vi "PathPlanner_TrigEventsSend.vi"(10 "Current Trig Events":T1[](array[typedef]) {"lastRobotPos"."Y" format="%14.3f"; "lastRobotPos"."X" format="%14.3f"; "markerPos"."Y" format="%14.3f"; "markerPos"."X" format="%14.3f"}) -> (2 "Past Trig EventMarkers":T1[](array[typedef]) {"lastRobotPos"."Y" format="%14.3f"; "lastRobotPos"."X" format="%14.3f"; "markerPos"."Y" format="%14.3f"; "markerPos"."X" format="%14.3f"}, 3 "Past Trig Events":string[](array[string]))   [LabVIEW 2023]
uses:
  <vilib>/Rock Robotics/WPI/ThirdParty/MJansen/PathPlanner/TypeDef/PathPlannerEventMarker.ctl
  <vilib>/Rock Robotics/WPI/ThirdParty/JAS_Junk/TrajLib/TypeDef/TRANSLATION2D.ctl
  <vilib>/Rock Robotics/WPI/ThirdParty/MJansen/PathPlanner/TypeDef/PathPlannerCommandUtil.ctl
  <vilib>/Rock Robotics/WPI/ThirdParty/MJansen/PathPlanner/ENum/PathPlanner_CommandUtilType_ENUM.ctl
  fee4c28f-3952-4fee-86c4-e7927070a504.vi
  <vilib>/Rock Robotics/WPI/ThirdParty/MJansen/PathPlanner/PathPlanner24.lvlib
  <vilib>/Rock Robotics/WPI/ThirdParty/JAS_Junk/TrajLib/Trajectory_Library.lvlib
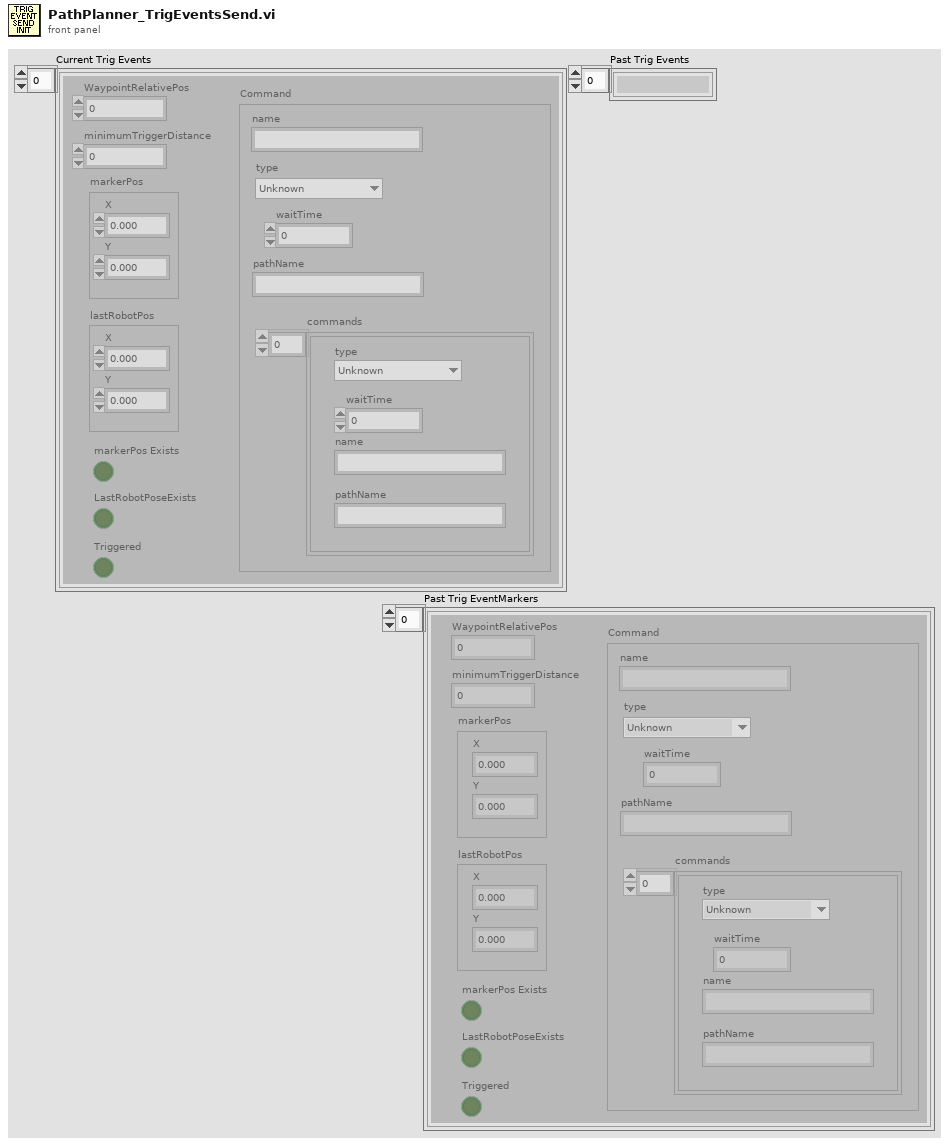
[diagram p1: front panel]
types:
  T1 = typedef "PathPlanner24.lvlib/PathPlannerEventMarker.ctl" = cluster{"WaypointRelativePos":dbl, "minimumTriggerDistance":dbl, "markerPos":T2, "lastRobotPos":T2, "Command":T3, "markerPos Exists":bool, "LastRobotPoseExists":bool, "Triggered":bool}
  T2 = typedef "Trajectory_Library.lvlib/TRANSLATION2D.ctl" = cluster{"X":dbl, "Y":dbl}
  T3 = typedef "PathPlanner24.lvlib/PathPlannerCommandUtil.ctl" = cluster{"waitTime":dbl, "name":string, "pathName":string, "commands":cluster{"type":T4, "waitTime":dbl, "name":string, "pathName":string}[], "type":T4}
  T4 = typedef "PathPlanner24.lvlib/PathPlanner_CommandUtilType_ENUM.ctl" = enum16{"Unknown", "Wait", "Named", "Path", "Sequential", "Parallel", "Race", "Deadline"}
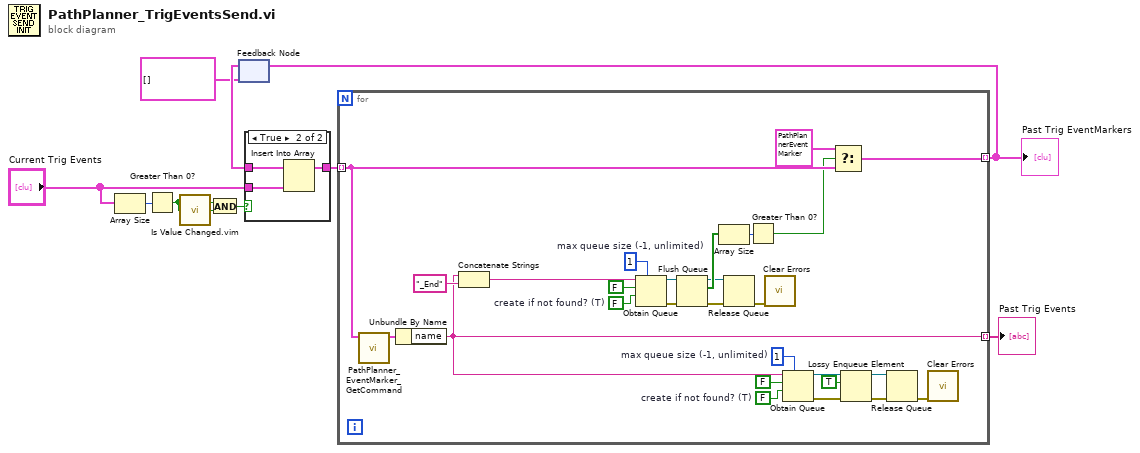
[diagram p0: block diagram]
diagram:
  n1 = Array Size(array="Current Trig Events") -> (size(s)=w3:i32)
  n2 = Greater Than 0?(x=w3) -> (x > 0?=w2:bool)
  n3 = call "Is Value Changed.vim"("value"=w2) -> ("changed or first call?"=w4:bool)
  n4 = And(x=w2, y=w4) -> (x .and. y?=w1:bool)
  n5 = feedback #1(T1[] []) -> (w10:T1[])
  n6 = case shown="True" w1 {
    tunnel: w10 -> [w11 w14]
    tunnel: "Current Trig Events" -> [_ w13]
    tunnel: [w11 w12] -> w7
    frame False {
    }
    frame True {
      n7 = Insert Into Array(array=w14, new element=w13) -> (w12:T1[])  [unwired: 1 in]
    }
  }
  n8 = for {
    tunnel: w7 -> [w18] mode=indexing
    tunnel: [w20] -> w8 mode=indexing
    tunnel: [w17] -> w6 mode=indexing
    w28 = FALSE  # create if not found? (T)
    w27 = 1  # max queue size (-1, unlimited)
    w36 = FALSE  # create if not found? (T)
    w32 = 1  # max queue size (-1, unlimited)
    n9 = call <vilib>:"PathPlanner_EventMarker_GetCommand.vi"("in EventMarker"=w18) -> ("Command"=w41:T3)  [unwired: 10 in]
    n10 = Unbundle By Name(w41) -> ("name"=w20:string)
    n11 = Concatenate Strings(w20, "_End" ("string")) -> (w19:string)
    n12 = Obtain Queue(max queue size (-1, unlimited)=w27, name (unnamed)=w19, element data type=FALSE, create if not found? (T)=w28) -> (queue out=w25:refnum<queue>, error out=w24:errorcluster)  [unwired: 1 in, 1 out]
    n13 = Flush Queue(queue=w25, error in (no error)=w24) -> (queue out=w23:refnum<queue>, remaining elements=w30:bool[], error out=w22:errorcluster)
    n14 = Array Size(array=w30) -> (size(s)=w31:i32)
    n15 = Release Queue(queue=w23, error in (no error)=w22) -> (error out=w26:errorcluster)  [unwired: 1 in, 2 out]
    n16 = Greater Than 0?(x=w31) -> (x > 0?=w15:bool)
    n17 = call <vilib>:"Clear Errors.vi"("error in (no error)"=w26) -> ()  [unwired: 5 in, 2 out]
    n18 = Obtain Queue(max queue size (-1, unlimited)=w32, name (unnamed)=w20, element data type=FALSE, create if not found? (T)=w36) -> (queue out=w39:refnum<queue>, error out=w40:errorcluster)  [unwired: 1 in, 1 out]
    n19 = Select(t=T1 {"WaypointRelativePos"=0.0, "minimumTriggerDistance"=0.0, "markerPos"={"X"=0.0, "Y"=0.0}, "lastRobotPos"={"X"=0.0, "Y"=0.0}, "Command"={"waitTime"=0.0, "name"="", "pathName"="", "commands"=[], "type"=enum."Unknown"}, "markerPos Exists"=FALSE, "LastRobotPoseExists"=FALSE, "Triggered"=FALSE}, s=w15, f=w18) -> (s? t:f=w17:T1)
    n20 = Lossy Enqueue Element(queue=w39, element=TRUE, error in (no error)=w40) -> (queue out=w33:refnum<queue>, error out=w35:errorcluster)  [unwired: 2 out]
    n21 = Release Queue(queue=w33, error in (no error)=w35) -> (error out=w34:errorcluster)  [unwired: 1 in, 2 out]
    n22 = call <vilib>:"Clear Errors.vi"("error in (no error)"=w34) -> ()  [unwired: 5 in, 2 out]
  }
  "Past Trig Events" <- w8
  "Past Trig EventMarkers" <- w6
  n23 = feedback-in #1(w6) -> ()
